vi "Protocolo_A.vi"(1 "Trama2":i8, 2 "Trama1":i8) -> (0 "Analogico":u32)   [LabVIEW 2017]
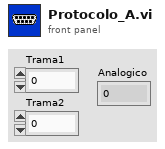
[diagram p1: front panel]
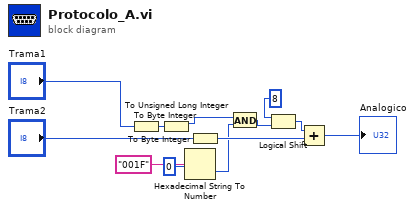
[diagram p0: block diagram]
diagram:
  n1 = To Byte Integer(number="Trama1") -> (8bit integer=w12:i8)
  n2 = To Unsigned Long Integer(number=w12) -> (unsigned 32bit integer=w5:u32)
  n3 = Hexadecimal String To Number(string="001F", offset=0) -> (number=w6:u32)  [unwired: 1 in, 1 out]
  n4 = To Byte Integer(number="Trama2") -> (8bit integer=w11:i8)
  n5 = And(x=w5, y=w6) -> (x .and. y?=w4:u32)
  n6 = Logical Shift(y=8, x=w4) -> (x << y=w9:u32)
  n7 = Add(x=w9, y=w11) -> (x+y=→"Analogico":u32)
